vi "Verify.vi"(7 "Test VI (caller)":string, 8 "error in (no error)":errorcluster, 10 "Test Data":string, 11 "LUnit Test Case In":refnum<class "Test Case.lvclass">) -> (0 "error out":errorcluster, 3 "LUnit Test Case Out":refnum<class "Test Case.lvclass">)   [LabVIEW 2020, in "LUnitExtension.lvlib"]
uses:
  LUnitExtension.lvlib
  <vilib>/Astemes/LUnit/Test Case.lvclass
  <vilib>/Astemes/LUnit/Test Case.lvclass/Test Case.ctl
  <vilib>/Astemes/LUnit/Append Fail Result.vi
  <vilib>/Astemes/LUnit/Append Pass Result.vi
  Approval Tests/Approval Tests.lvlib
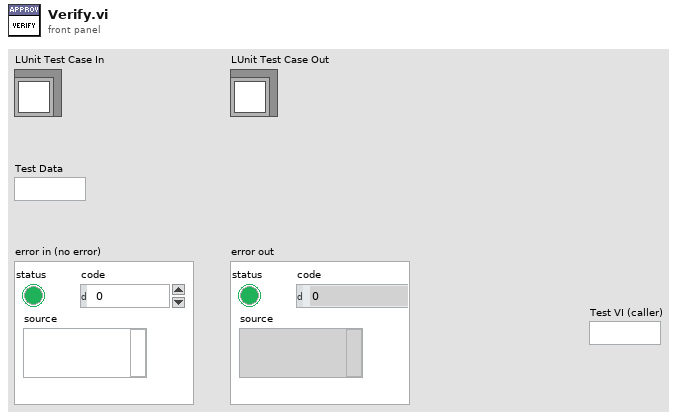
[diagram p1: front panel]
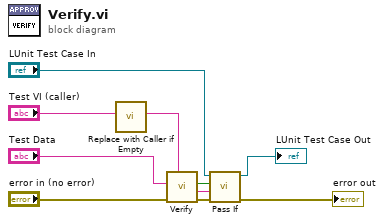
[diagram p0: block diagram]
diagram:
  n1 = call "Replace with Caller if Empty.vi"("Test VI (caller) in"="Test VI (caller)") -> ("Test VI (caller) out"=w1:string)  [unwired: 10 in]
  n2 = call "Verify.vi"("Test VI (caller)"=w1, "error in"="error in (no error)", "Test Data"="Test Data") -> ("error out"=w6:errorcluster, "Failure Message"=w3:string, "Passed?"=w4:bool)  [unwired: 6 in]
  n3 = call <vilib>:"Pass If.vi"("error in (no error)"=w6, "Message"=w3, "Pass?"=w4, "LUnit Test Case In"="LUnit Test Case In") -> ("error out"=→"error out":errorcluster, "LUnit Test Case Out"=→"LUnit Test Case Out":refnum<class "Test Case.lvclass">)  [unwired: 6 in]
